vi "[GV]_GPS Checksum.vi"() -> ()   [LabVIEW 2016]
panel:
  out "GPS Checksum":bool
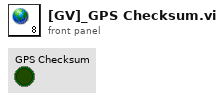
[diagram p1: front panel]
diagram:
